vi "H036 Harsh Pandit SCADA Lab 4b Sem 6.vi"() -> ()   [LabVIEW 2018]
panel:
  out "Waveform Chart":dbl(graph)
  in  "Frequency":dbl(knob) scale=0.0..5.0
  in  "Amplitude":dbl(knob) scale=0.0..20.0
  # "Experiment 4b: Develope sine wave generator using while loop. Vary the amplitude and frequency using knob"
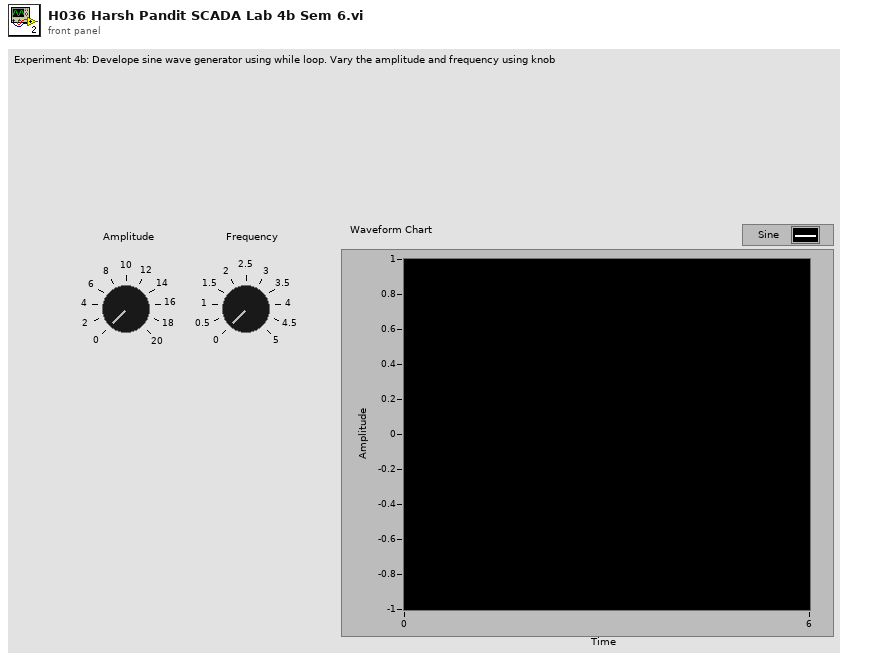
[diagram p1: front panel]
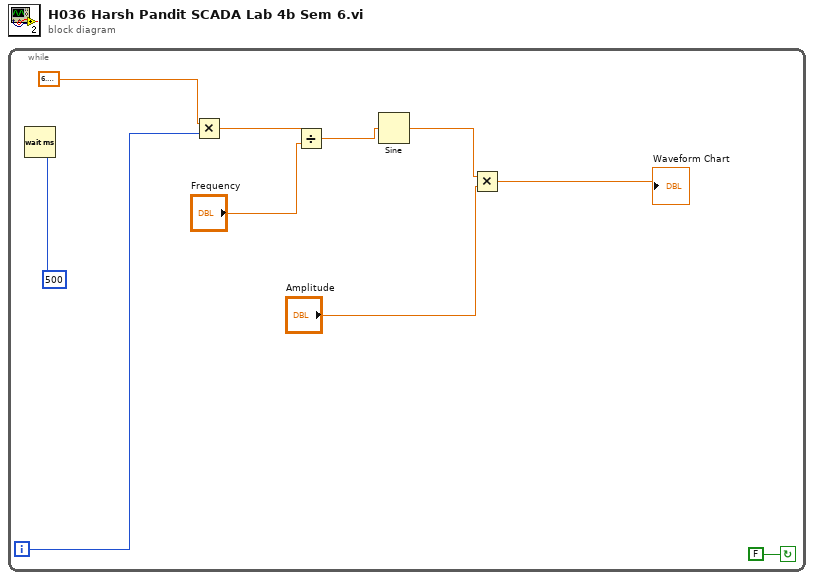
[diagram p0: block diagram]
diagram:
  n1 = while {
    i -> [w2]
    stop <- FALSE continue-if-true
    n2 = Wait (ms)(milliseconds to wait=500) -> ()  [unwired: 1 out]
    n3 = Multiply(x=6.283185307179586, y=w2) -> (x*y=w4:dbl)
    n4 = Divide(x=w4, y="Frequency") -> (x/y=w6:dbl)
    n5 = Sine(x=w6) -> (sin(x)=w10:dbl)
    n6 = Multiply(x=w10, y="Amplitude") -> (x*y=→"Waveform Chart":dbl)
  }
